vi "BRAM U64_Xilinx.vi"(0 "Address 0":fxp<+,11,11>, 1 "Address0.Data":u64, 2 "Address0.Write?":bool, 3 "Address 1":fxp<+,11,11>, 4 "Address 1.Data":u64, 5 "Address1 Write?":bool) -> (15 "Address 0.Element":u64, 18 "Address 1.Element":u64)   [LabVIEW 2011]
uses:
  <vilib>/rvi/IPIntegrationNode/IPINode_Utilities/niFpgaIPINodeSimCore.vi
  <vilib>/rvi/XilinxIP/XIPIN_XNode/niFpgaXIPIN.xnode
  <userlib>/FPGA Library/Code Development/BRAM/Xilinx BRAM U64/Core/BRAMU64_B53F670C470B51929A8281862D9F4557.dll
  <vilib>/rvi/IPIntegrationNode/IPINode_Xnode/niFpgaIPINode.xnode
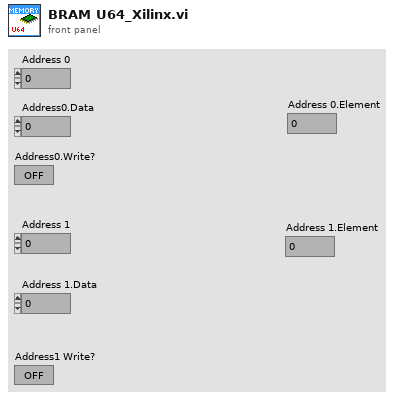
[diagram p1: front panel]
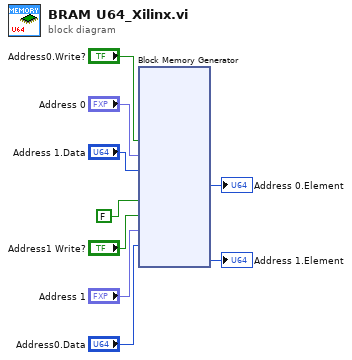
[diagram p0: block diagram]
diagram:
  n1 = xnode ("Block Memory Generator")("wea"="Address0.Write?", "addra"="Address 0", "dina"="Address 1.Data", "clkb"=FALSE, "web"="Address1 Write?", "addrb"="Address 1", "dinb"="Address0.Data") -> ("douta"=→"Address 0.Element":u64, "doutb"=→"Address 1.Element":u64)
